vi "Read String Convert.vi"(8 "error in":errorcluster, 10 "read string in":string) -> (0 "error out":errorcluster, 2 "4position":i32[](array[numeric]), 3 "read string out":string)   [LabVIEW 2019, in "Allmotion.lvlib"]
uses:
  Allmotion.lvlib
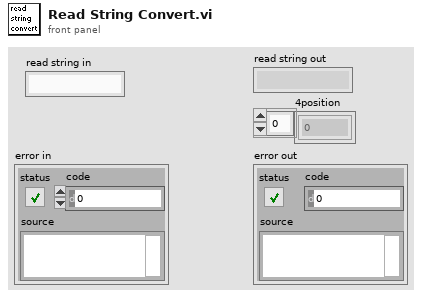
[diagram p1: front panel]
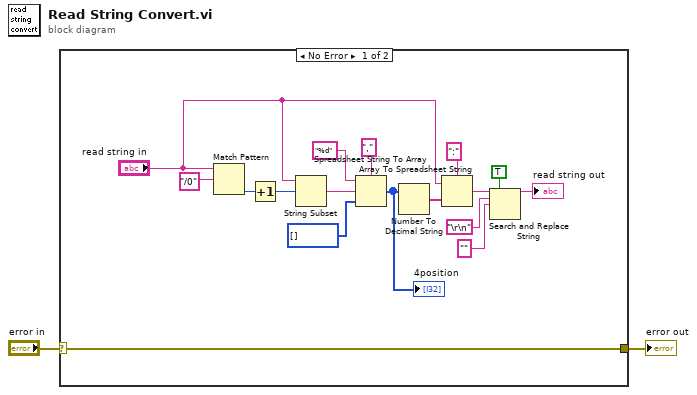
[diagram p0: block diagram]
diagram:
  n1 = case shown="No Error" "error in" {
    selector: "error in" -> [w3 w20]
    tunnel: [w3 w20] -> w1
    frame No Error {
      n2 = Match Pattern(string="read string in", regular expression="/0") -> (offset past match=w18:i32)  [unwired: 1 in, 3 out]
      n3 = Increment(x=w18) -> (x+1=w17:i32)
      n4 = String Subset(string="read string in", offset (0)=w17) -> (substring=w16:string)  [unwired: 1 in]
      n5 = Spreadsheet String To Array(delimiter (Tab)=",", format string="%d", spreadsheet string=w16, array type (2D Dbl)=i32[] []) -> (array=w7:i32[])
      "4position" <- w7
      n6 = Number To Decimal String(number=w7) -> (decimal integer string=w12:string[])  [unwired: 1 in]
      n7 = Array To Spreadsheet String(delimiter (Tab)=":", array=w12, 3:"read string in") -> (spreadsheet string=w5:string)
      n8 = Search and Replace String(replace all?=TRUE ("replace all? (F)"), input string=w5, search string="\r\n", replace string="" ("replace string (\"\")")) -> (result string=→"read string out":string)  [unwired: 4 in, 3 out]
    }
    frame Error {
    }
  }
  "error out" <- w1
